vi "Update Source Count.vi"(8 "error in (no error)":errorcluster, 11 "BuildSpec in":refnum<vi>) -> (0 "error out":errorcluster, 3 "BuildSpec out":refnum<vi>)   [LabVIEW 2019, in "Project Sync Tools.lvclass"]
uses:
  Project Sync Tools.lvclass
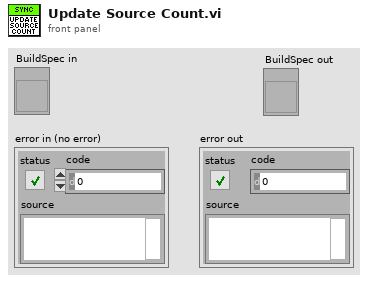
[diagram p1: front panel]
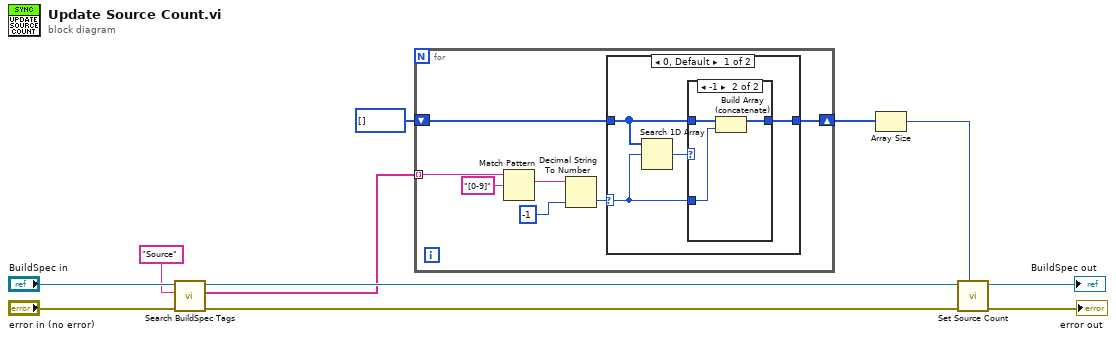
[diagram p0: block diagram]
diagram:
  n1 = call "Search BuildSpec Tags.vi"("error in (no error)"="error in (no error)", "Regular expression"="Source", "BuildSpec in"="BuildSpec in") -> ("error out"=w8:errorcluster, "Tag Names"=w3:string[], "BuildSpec out"=w9:refnum<vi>)  [unwired: 6 in]
  n2 = for {
    tunnel: w3 -> [w18] mode=indexing
    shift-right: [w13] -> w5
    shift-left: i32[] [] -> [w14]
    n3 = Match Pattern(string=w18, regular expression="[0-9]") -> (match substring=w16:string)  [unwired: 1 in, 3 out]
    n4 = Decimal String To Number(string=w16, default (0L)=-1 ("default (0 I32)")) -> (number=w12:i32)  [unwired: 1 in, 1 out]
    n5 = case shown="0, Default" w12 {
      selector: w12 -> [w19 _]
      tunnel: w14 -> [w21 w27]
      tunnel: [w20 w27] -> w13
      frame 0, Default {
        n6 = Search 1D Array(1D array=w21, element=w19) -> (index of element=w22:i32)  [unwired: 1 in]
        n7 = case shown="-1" w22 {
          tunnel: w21 -> [w23 w26]
          tunnel: w19 -> [_ w25]
          tunnel: [w23 w24] -> w20
          frame 0, Default {
          }
          frame -1 {
            n8 = Build Array (concatenate)(w26, w25) -> (w24:i32[])
          }
        }
      }
      frame -1 {
      }
    }
  }
  n9 = Array Size(array=w5) -> (size(s)=w11:i32)
  n10 = call "Set Source Count.vi"("Source Count"=w11, "error in (no error)"=w8, "BuildSpec in"=w9) -> ("error out"=→"error out":errorcluster, "BuildSpec out"=→"BuildSpec out":refnum<vi>)  [unwired: 7 in]
